vi "magnitude_of_acceleration_vectors.vi"(8 "error in":errorcluster, 11 "all in one package in":T1 {"time informations"."length" format="%<%H:%M:%S%3u>t"; "actigraph settings"."id" format="%02d"; "actigraph settings"."range code" format="%02x"; "actigraph settings"."rate code" format="%02x"}) -> (0 "error out":errorcluster, 3 "all in one package out":T1 {"time informations"."length" format="%<%H:%M:%S%3u>t"; "actigraph settings"."id" format="%02d"; "actigraph settings"."range code" format="%02x"; "actigraph settings"."rate code" format="%02x"})   [LabVIEW 2017]
uses:
  Controls/gyro_control_memory_structure.ctl
  Controls/gyro_control_measurement_settings.ctl
  Controls/gyro_control_time_informations.ctl
  Controls/gyro_control_measurement_data.ctl
  Controls/gyro_control_all_in_one_package.ctl
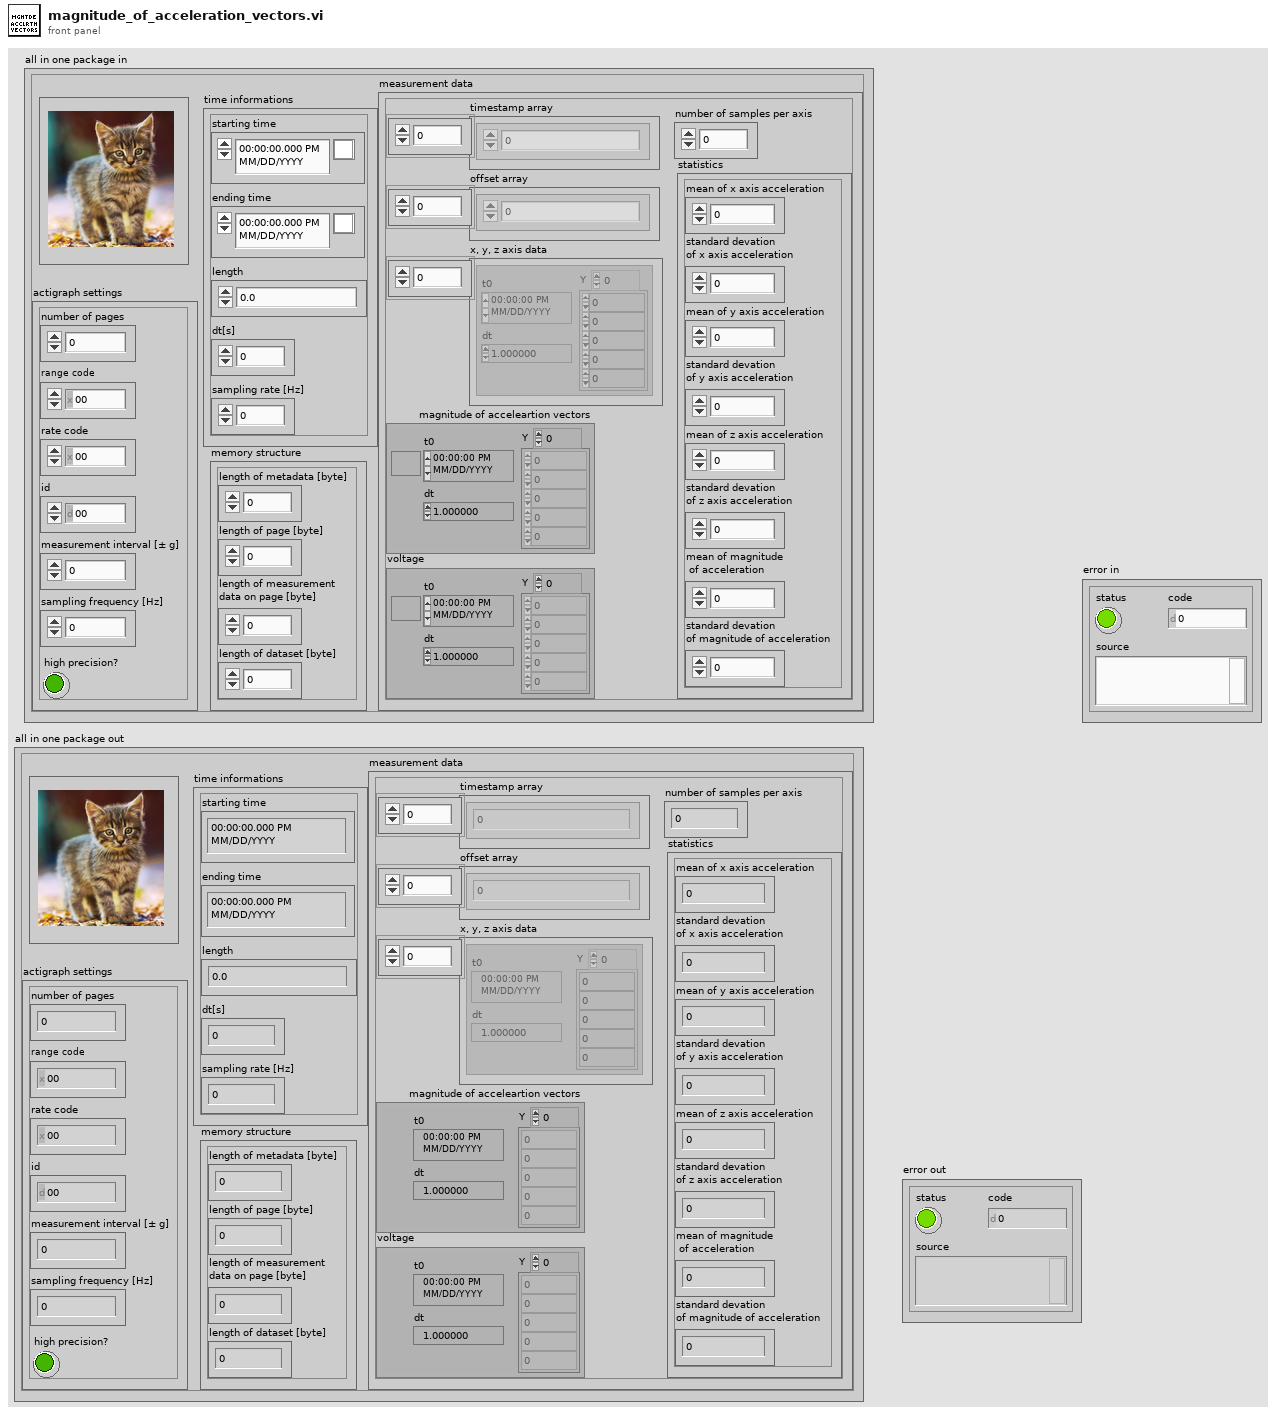
[diagram p1: front panel]
types:
  T1 = typedef "gyro_control_all_in_one_package.ctl" = cluster{"measurement data":T2, "actigraph settings":T3, "memory structure":T4, "time informations":T5}
  T2 = typedef "gyro_control_measurement_data.ctl" = cluster{"number of samples per axis":i32, "timestamp array":dbl[], "offset array":dbl[], "x, y, z axis data":waveform(dbl)[], "magnitude of acceleartion vectors":waveform(dbl), "statistics":cluster{"mean of x axis acceleration":dbl, "standard devation \nof x axis acceleration":dbl, "mean of y axis acceleration":dbl, "standard devation \nof y axis acceleration":dbl, "mean of z axis acceleration":dbl, "standard devation \nof z axis acceleration":dbl, "mean of magnitude\n of acceleration":dbl, "standard devation \nof magnitude of acceleration":dbl}, "voltage":waveform(dbl)}
  T3 = typedef "control_measurement_settings.ctl" = cluster{"sampling frequency [Hz]":dbl, "measurement interval [± g]":i32, "high precision?":bool, "number of pages":i32, "rate code":i32, "range code":i32, "id":i32}
  T4 = typedef "gyro_control_memory_structure.ctl" = cluster{"length of metadata [byte]":i32, "length of page [byte]":i32, "length of measurement \ndata on page [byte]":i32, "length of dataset [byte]":i32}
  T5 = typedef "gyro_control_time_informations.ctl" = cluster{"starting time":timestamp, "ending time":timestamp, "dt[s]":dbl, "sampling rate [Hz]":dbl, "length":dbl}
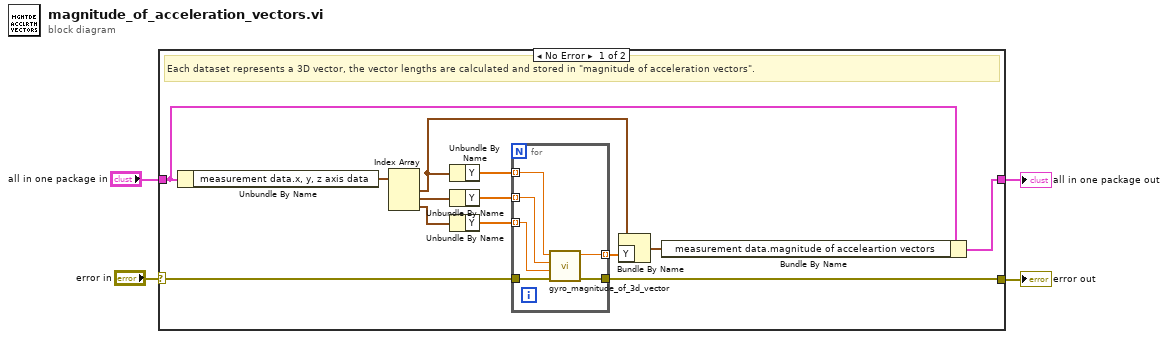
[diagram p0: block diagram]
diagram:
  n1 = case shown="No Error" "error in" {
    selector: "error in" -> [w11 w24]
    tunnel: [w10 w24] -> w3
    tunnel: "all in one package in" -> [w7 w25]
    tunnel: [w5 w25] -> w1
    frame No Error {
      # "Each dataset represents a 3D vector, the vector lengths are calculated and stored in \"magnitude of acceleration vectors\"."
      n2 = Unbundle By Name(w7) -> ("measurement data.x, y, z axis data"=w17:waveform(dbl)[])
      n3 = Index Array(array=w17) -> (element #1=w8:waveform(dbl), element #2=w16:waveform(dbl), element #3=w15:waveform(dbl))  [unwired: 3 in]
      n4 = Unbundle By Name(w8) -> ("Y"=w14:dbl[])
      n5 = Unbundle By Name(w16) -> ("Y"=w13:dbl[])
      n6 = Unbundle By Name(w15) -> ("Y"=w12:dbl[])
      n7 = for {
        tunnel: w14 -> [w21] mode=indexing
        tunnel: w13 -> [w20] mode=indexing
        tunnel: w12 -> [w19] mode=indexing
        tunnel: w11 -> [w23]
        tunnel: [w22] -> w10
        tunnel: [w18] -> w9 mode=indexing
        n8 = call "gyro_magnitude_of_3d_vector.vi"("error in"=w23, "z axis component"=w19, "y axis component"=w20, "x axis component"=w21) -> ("error out"=w22:errorcluster, "magnitude of 3d vector"=w18:dbl)  [unwired: 6 in]
      }
      n9 = Bundle By Name(cluster=w8, "Y"=w9) -> (w6:waveform(dbl))
      n10 = Bundle By Name(cluster=w7, "measurement data.magnitude of acceleartion vectors"=w6) -> (w5:T1)
    }
    frame Error {
    }
  }
  "error out" <- w3
  "all in one package out" <- w1
